vi "StarCount.vi"(1 "Boolean 2":bool, 2 "Boolean":bool, 3 "Boolean 3":bool) -> (0 "Numeric":dbl)   [LabVIEW 2014]
panel:
  in  "Array":bool[](array[boolean])
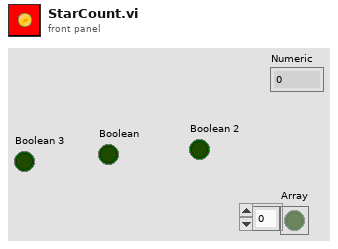
[diagram p1: front panel]
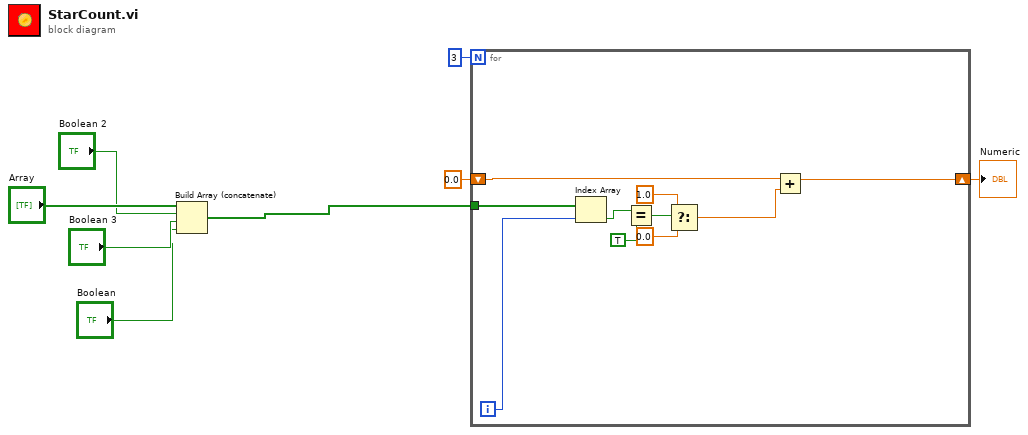
[diagram p0: block diagram]
diagram:
  n1 = Build Array (concatenate)("Array", "Boolean 2", "Boolean 3", "Boolean") -> (w3:bool[])
  n2 = for {
    N: 3 -> [_]
    tunnel: w3 -> [w18]
    shift-right: [w12] -> w1
    shift-left: 0.0 -> [w13]
    i -> [w17]
    n3 = Index Array(array=w18, index=w17) -> (element=w16:bool)
    n4 = Equal?(x=w16, y=TRUE) -> (x = y?=w14:bool)
    n5 = Select(t=1.0, s=w14, f=0.0) -> (s? t:f=w9:dbl)
    n6 = Add(x=w13, y=w9) -> (x+y=w12:dbl)
  }
  "Numeric" <- w1
